vi "Configure Standard Waveform.vi"(4 "Frequency (1000.0 Hz)":dbl=1000.0, 6 "DC Offset (0.0 Volts)":dbl, 7 "Waveform (0: Sine)":u16(ring) items=["Sine", "Square", "Ramp Up", "Ramp Down", "Pulse", "Noise", "DC"], 8 "error in (no error)":errorcluster, 9 "Amplitude (1.0 Vpp)":dbl=1.0, 10 "Channel (1: Channel1)":u16(ring)=1 items=["Channel1"=1, "Channel2"=2], 11 "VISA resource name":refnum<visa-resource-name>) -> (0 "error out":errorcluster, 3 "VISA resource name out":refnum<visa-resource-name>)   [LabVIEW 2009, in "Agilent 81150.lvlib"]
doc: "Selects the waveform shape, frequency, amplitude, offset, and phase for a standard waveform."
uses:
  Agilent 81150.lvlib
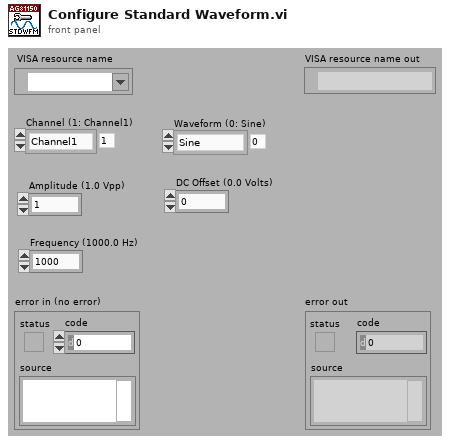
[diagram p1: front panel]
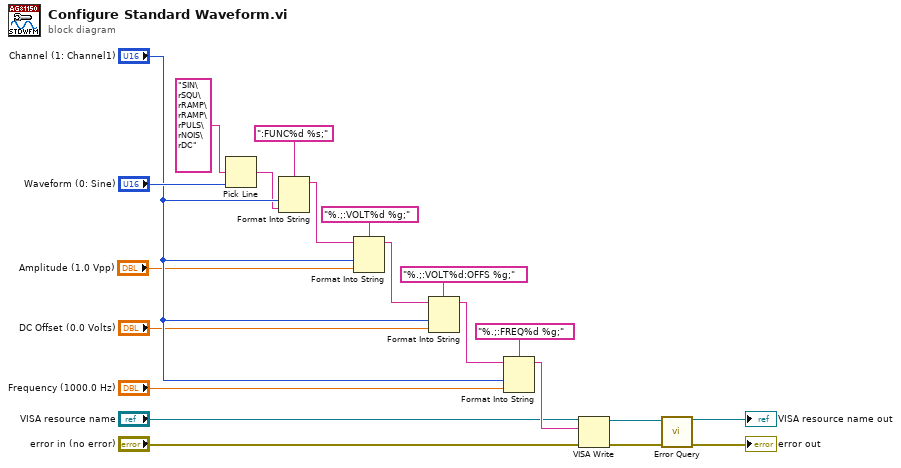
[diagram p0: block diagram]
diagram:
  n1 = Pick Line(multi-line string="SIN\rSQU\rRAMP\rRAMP\rPULS\rNOIS\rDC", line index="Waveform (0: Sine)") -> (output string=w17:string)  [unwired: 1 out]
  n2 = Format Into String(format string=":FUNC%d %s;", "Channel (1: Channel1)", w17) -> (resulting string=w15:string)  [unwired: 2 in, 1 out]
  n3 = Format Into String(format string="%.;:VOLT%d %g;", initial string=w15, "Channel (1: Channel1)", "Amplitude (1.0 Vpp)") -> (resulting string=w12:string)  [unwired: 1 in, 1 out]
  n4 = Format Into String(format string="%.;:VOLT%d:OFFS %g;", initial string=w12, "Channel (1: Channel1)", "DC Offset (0.0 Volts)") -> (resulting string=w9:string)  [unwired: 1 in, 1 out]
  n5 = Format Into String(format string="%.;:FREQ%d %g;", initial string=w9, "Channel (1: Channel1)", "Frequency (1000.0 Hz)") -> (resulting string=w7:string)  [unwired: 1 in, 1 out]
  n6 = VISA Write(VISA resource name="VISA resource name", write buffer=w7, error in (no error)="error in (no error)") -> (VISA resource name out=w4:refnum<visa-resource-name>, error out=w3:errorcluster)  [unwired: 1 out]
  n7 = call "Error Query.vi"("error in (no error)"=w3, "VISA resource name"=w4) -> ("error out"=→"error out":errorcluster, "VISA resource name out"=→"VISA resource name out":refnum<visa-resource-name>)  [unwired: 8 out]
